vi "repeat cycle_linear down.vi"(8 "error in (no error)":errorcluster caption="에러 입력(에러 없음)", 10 "waveform in":waveform(dbl), 11 "Waveform Obj 입력":refnum<class "Waveform Gen.lvclass">) -> (0 "error out":errorcluster caption="에러 출력", 2 "waveform out":waveform(dbl), 3 "Waveform Obj 출력":refnum<class "Waveform Gen.lvclass">)   [LabVIEW 2020, in "Waveform Gen.lvclass"]
uses:
  Waveform Gen.lvclass
  Waveform Gen.lvclass/Waveform Gen.ctl
  Accessors/Read cycle.vi
  <vilib>/Waveform/WDTOps.llb/WDT Append Waveforms DBL.vi
  <vilib>/Waveform/WDTOps.llb/WDT Number of Waveform Samples DBL.vi
  <vilib>/Waveform/WDTOps.llb/WDT Get Waveform Subset DBL.vi
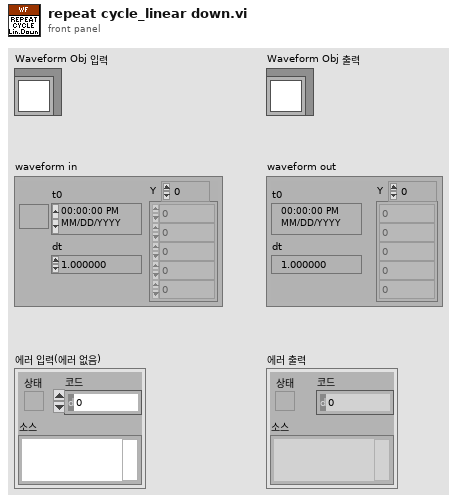
[diagram p1: front panel]
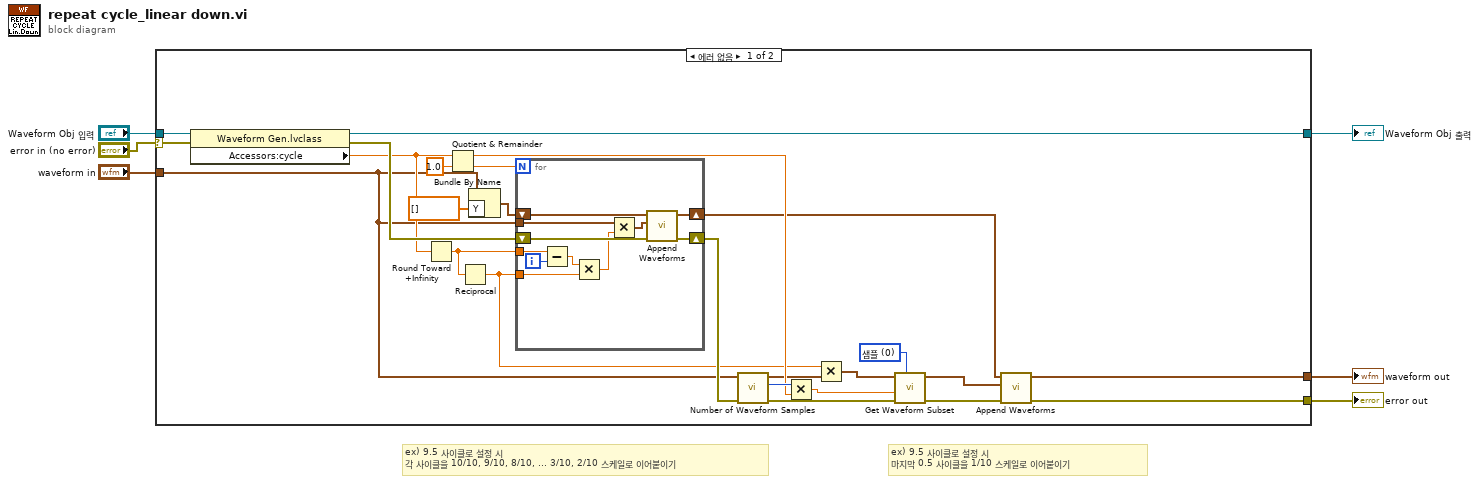
[diagram p0: block diagram]
diagram:
  # "ex) 9.5 사이클로 설정 시 \n마지막 0.5 사이클을 1/10 스케일로 이어붙이기"
  # "ex) 9.5 사이클로 설정 시 \n각 사이클을 10/10, 9/10, 8/10, ... 3/10, 2/10 스케일로 이어붙이기"
  n1 = case shown="에러 없음" "error in (no error)" {
    selector: "error in (no error)" -> [w29 w44]
    tunnel: [w8 w44] -> w3
    tunnel: "Waveform Obj 입력" -> [w31 w43]
    tunnel: [w9 w43] -> w5
    tunnel: "waveform in" -> [w10 _]
    tunnel: [w7 _] -> w1
    frame No Error {
      w18 = u16 0 items=["샘플", "상대 시간"] ("start/duration format")
      n2 = property class="Waveform Gen.lvclass"(reference=w31, error in=w29) -> (reference out=w9:refnum<class "Waveform Gen.lvclass">, error out=w22:errorcluster, "Accessors:cycle"=w17:dbl)
      n3 = Round Toward +Infinity(x=w17) -> (ceil(x): smallest int >= x=w14:dbl)
      n4 = Quotient & Remainder(x=w17, y=1.0) -> (x-y*floor(x/y)=w26:dbl, floor(x/y)=w28:dbl)
      n5 = Reciprocal(x=w14) -> (1/x=w15:dbl)
      n6 = Bundle By Name(cluster=w10, "Y"=dbl[] []) -> (w11:waveform(dbl))
      n7 = for {
        N: w28 -> [_]
        shift-right: [w41] -> w13
        shift-left: w11 -> [w42]
        shift-right: [w39] -> w21
        shift-left: w22 -> [w40]
        tunnel: w10 -> [w38]
        tunnel: w14 -> [w37]
        tunnel: w15 -> [w34]
        i -> [w36]
        n8 = Subtract(x=w37, y=w36) -> (x-y=w35:dbl)
        n9 = Multiply(x=w35, y=w34) -> (x*y=w32:dbl)
        n10 = Multiply(x=w38, y=w32) -> (x*y=w33:waveform(dbl))
        n11 = call-poly <vilib>:"Append Waveforms.vi"("error in (no error)"=w40, "waveform B"=w33, "waveform A"=w42) -> ("error out"=w39:errorcluster, "waveform out"=w41:waveform(dbl))  [unwired: 7 in]
      }
      n12 = call-poly <vilib>:"Number of Waveform Samples.vi"("error in (no error)"=w21, "waveform in"=w10) -> ("error out"=w24:errorcluster, "number of samples"=w27:i32, "waveform out"=w19:waveform(dbl))  [unwired: 7 in]
      n13 = Multiply(x=w27, y=w26) -> (x*y=w25:dbl)
      n14 = Multiply(x=w15, y=w19) -> (x*y=w16:waveform(dbl))
      n15 = call-poly <vilib>:"Get Waveform Subset.vi"("start/duration format"=w18, "error in (no error)"=w24, "duration"=w25, "waveform in"=w16) -> ("error out"=w20:errorcluster, "waveform out"=w23:waveform(dbl))  [unwired: 2 in, 2 out]
      n16 = call-poly <vilib>:"Append Waveforms.vi"("error in (no error)"=w20, "waveform B"=w23, "waveform A"=w13) -> ("error out"=w8:errorcluster, "waveform out"=w7:waveform(dbl))  [unwired: 7 in]
    }
    frame Error {
    }
  }
  "error out" <- w3
  "Waveform Obj 출력" <- w5
  "waveform out" <- w1
